vi "首页显示设置.vi"() -> ()   [LabVIEW 2016]
uses:
  <vilib>/Utility/miscctls.llb/LVPointTypeDef.ctl
  <vilib>/Utility/config.llb/NI_LVConfig.lvlib
panel:
  in  "CODCr":bool caption="氨氮禁用"
  in  "ORP":bool caption="氨氮禁用"
  in  "硫化物":bool caption="氨氮禁用"
  in  "亚硝氮":bool caption="氨氮禁用"
  in  "硝氮":bool caption="氨氮禁用"
  in  "确认":bool
  in  "藻密度":bool=TRUE caption="氨氮禁用"
  in  "叶绿素a":bool=TRUE caption="氨氮禁用"
  in  "湿度":bool=TRUE caption="氨氮禁用"
  in  "室温":bool=TRUE caption="氨氮禁用"
  in  "电压":bool=TRUE caption="氨氮禁用"
  in  "CODMn":bool=TRUE caption="氨氮禁用"
  in  "总氮":bool=TRUE caption="氨氮禁用"
  in  "总磷":bool=TRUE caption="氨氮禁用"
  in  "氨氮":bool=TRUE caption="氨氮禁用"
  in  "Turb":bool=TRUE caption="氨氮禁用"
  in  "Cond":bool=TRUE caption="氨氮禁用"
  in  "DO":bool=TRUE caption="氨氮禁用"
  in  "pH":bool=TRUE caption="氨氮禁用"
  in  "水温":bool=TRUE caption="氨氮禁用"
  # "请选择首页要显示的参数"
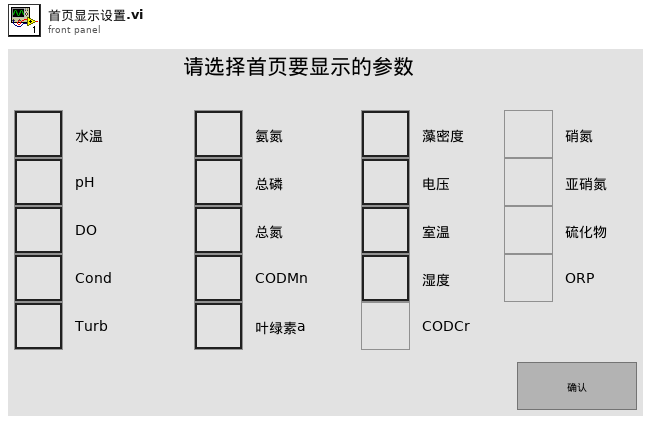
[diagram p1: front panel]
types:
  T1 = typedef "LVPointTypeDef.ctl" = cluster{"Horizontal":i16, "Vertical":i16}
  T2 = typedef "NI_LVConfig.lvlib/Config Data RefNum.ctl" = refnum<k1>
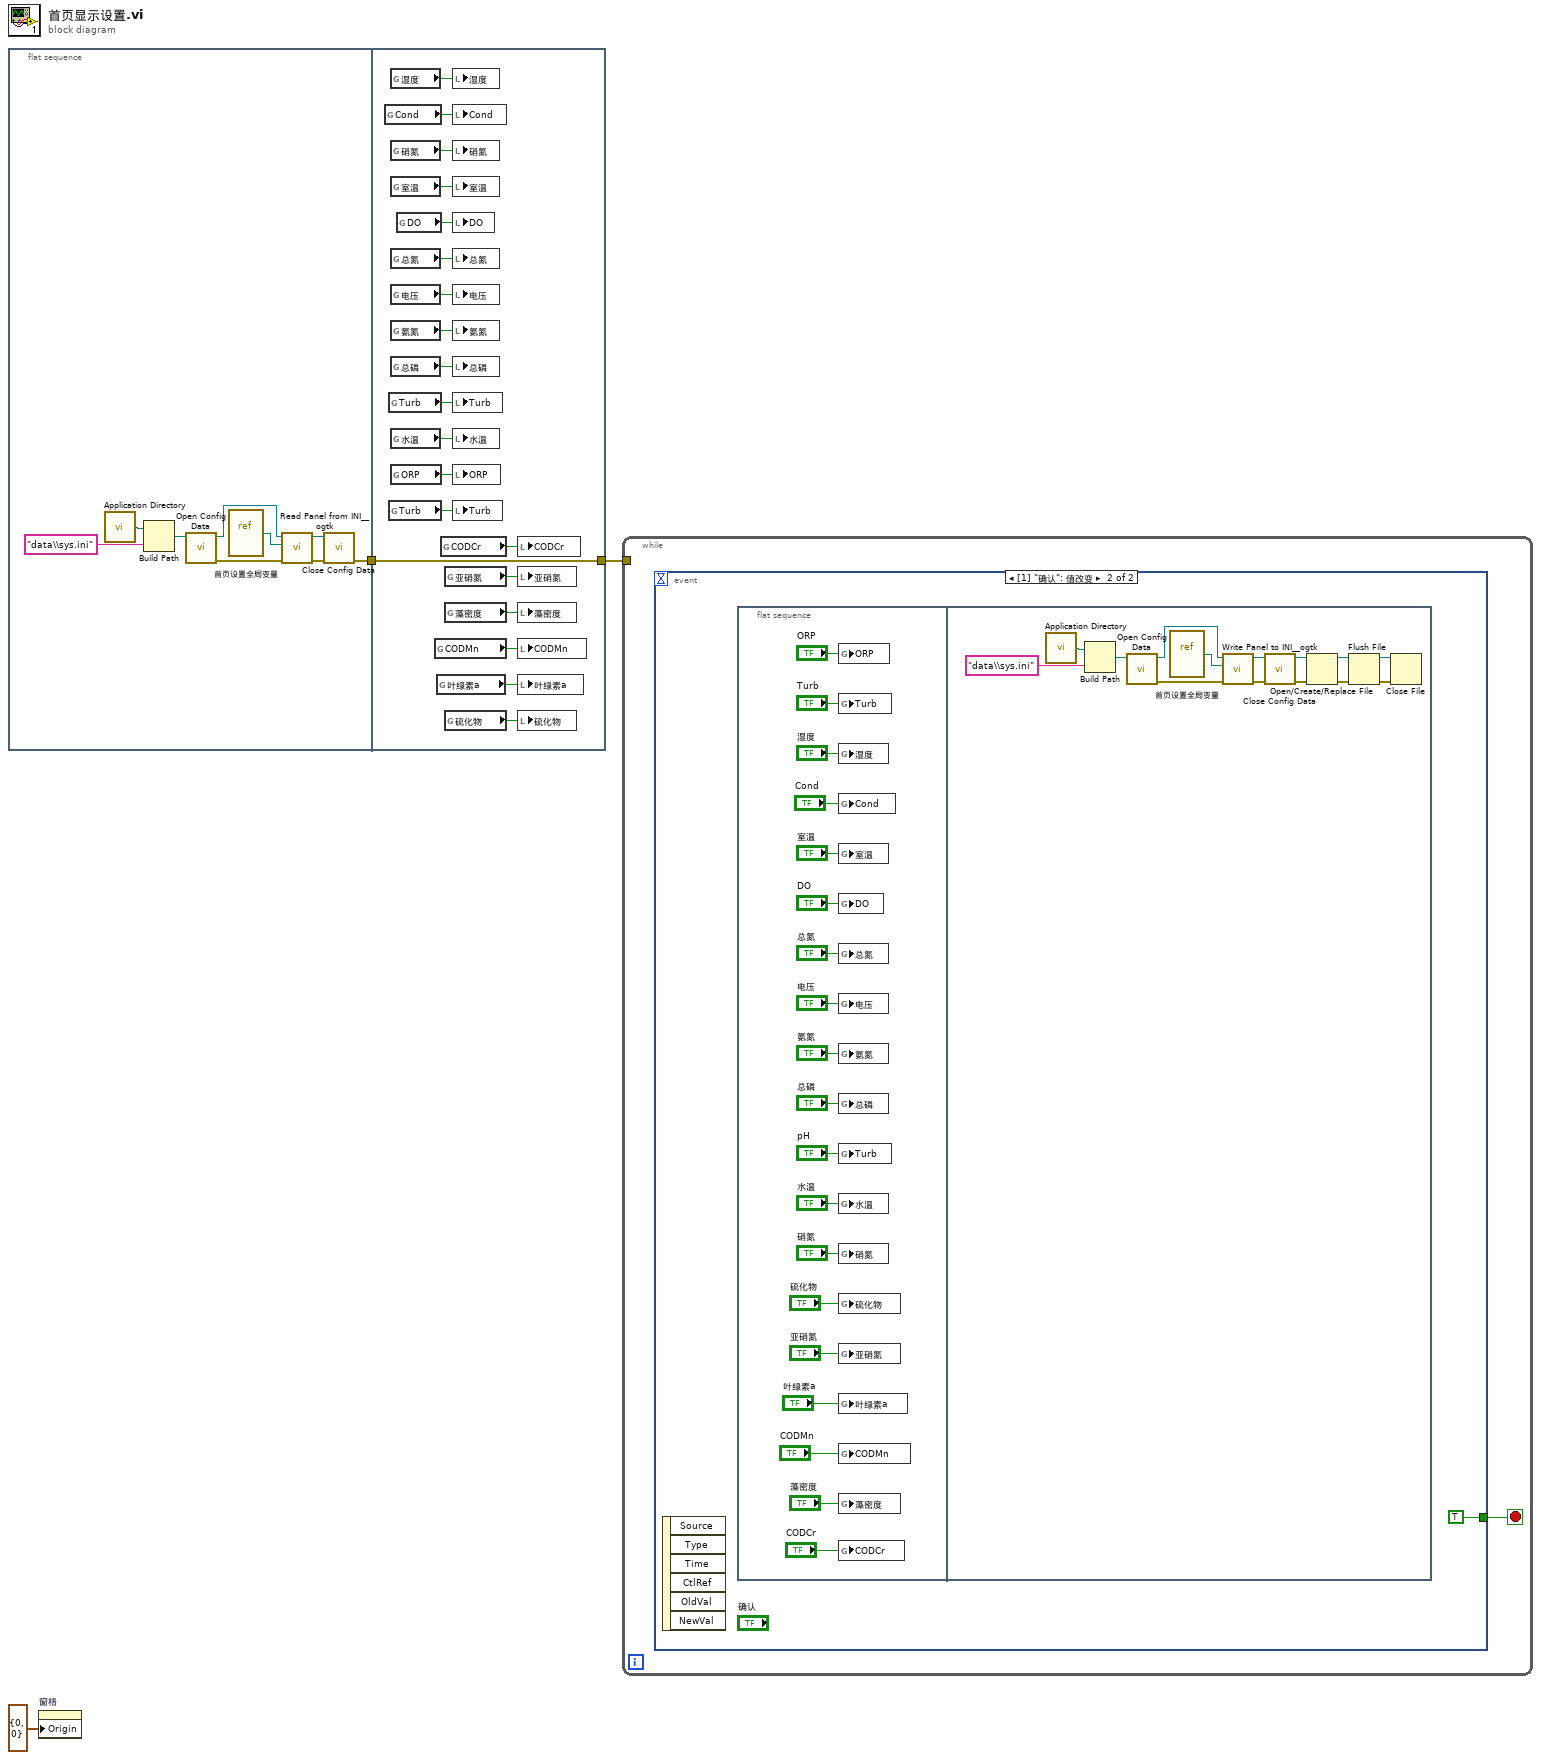
[diagram p0: block diagram]
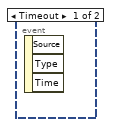
[diagram p2: hidden frame]
diagram:
  n1 = flat-sequence {
    tunnel: [w4] -> w2
    tunnel: w2 -> [w18]
    tunnel: [w18] -> w1
    frame #0 {
      n2 = call <vilib>:"Application Directory.vi"() -> ("Application Directory"=w12:path)
      n3 = Build Path(base path=w12, name or relative path="data\\sys.ini" ("名称或相对路径")) -> (appended path=w10:path)
      n4 = call <vilib>:"Open Config Data.vi"("configuration file path"=w10) -> ("error out"=w6:errorcluster, "refnum"=w9:T2)  [unwired: 8 in, 1 out]
      n5 = vi-ref "首页设置全局变量.vi"() -> (w8:refnum<vi>)
      n6 = call <userlib>:"Read Panel from INI__ogtk.vi"("error in (no error)"=w6, "VI ref"=w8, "refnum"=w9) -> ("error out"=w5:errorcluster, "refnum out"=w7:T2)  [unwired: 7 in]
      n7 = call <vilib>:"Close Config Data.vi"("error in (no error)"=w5, "refnum"=w7) -> ("error out"=w4:errorcluster)  [unwired: 8 in, 1 out]
    }
    frame #1 {
      n8 = global read "首页设置全局变量.vi" "Cond"() -> (w19:bool)
      n9 = global read "首页设置全局变量.vi" "Turb"() -> (w26:bool)
      n10 = global read "首页设置全局变量.vi" "Turb"() -> (w28:bool)
      n11 = global read "首页设置全局变量.vi" "湿度"() -> (w32:bool)
      n12 = global read "首页设置全局变量.vi" "硝氮"() -> (w17:bool)
      n13 = global read "首页设置全局变量.vi" "室温"() -> (w20:bool)
      n14 = global read "首页设置全局变量.vi" "总氮"() -> (w22:bool)
      n15 = global read "首页设置全局变量.vi" "电压"() -> (w23:bool)
      n16 = global read "首页设置全局变量.vi" "氨氮"() -> (w24:bool)
      n17 = global read "首页设置全局变量.vi" "总磷"() -> (w25:bool)
      n18 = global read "首页设置全局变量.vi" "水温"() -> (w27:bool)
      n19 = global read "首页设置全局变量.vi" "ORP"() -> (w14:bool)
      n20 = global read "首页设置全局变量.vi" "DO"() -> (w21:bool)
      n21 = global read "首页设置全局变量.vi" "CODMn"() -> (w30:bool)
      n22 = global read "首页设置全局变量.vi" "叶绿素a"() -> (w29:bool)
      n23 = global read "首页设置全局变量.vi" "CODCr"() -> (w13:bool)
      n24 = global read "首页设置全局变量.vi" "亚硝氮"() -> (w16:bool)
      n25 = global read "首页设置全局变量.vi" "藻密度"() -> (w31:bool)
      n26 = global read "首页设置全局变量.vi" "硫化物"() -> (w15:bool)
      n27 = local write "湿度"(w32) -> ()
      n28 = local write "Cond"(w19) -> ()
      n29 = local write "硝氮"(w17) -> ()
      n30 = local write "室温"(w20) -> ()
      n31 = local write "DO"(w21) -> ()
      n32 = local write "总氮"(w22) -> ()
      n33 = local write "电压"(w23) -> ()
      n34 = local write "氨氮"(w24) -> ()
      n35 = local write "总磷"(w25) -> ()
      n36 = local write "Turb"(w26) -> ()
      n37 = local write "水温"(w27) -> ()
      n38 = local write "ORP"(w14) -> ()
      n39 = local write "Turb"(w28) -> ()
      n40 = local write "CODCr"(w13) -> ()
      n41 = local write "亚硝氮"(w16) -> ()
      n42 = local write "藻密度"(w31) -> ()
      n43 = local write "CODMn"(w30) -> ()
      n44 = local write "叶绿素a"(w29) -> ()
      n45 = local write "硫化物"(w15) -> ()
    }
  }
  n46 = property on="窗格" class="Pane"("Origin"=T1 {"Horizontal"=0, "Vertical"=0} ("原点")) -> ()  [unwired: 2 in, 2 out]
  n47 = while {
    tunnel: w1 -> [_]
    stop <- w33 stop-if-true
    n48 = event shown="[1] \"确认\": 值改变" {
      selector: _ -> [_ _]
      dyn-events: _ -> [_ _]
      timeout: _ -> [_ _]
      tunnel: [_ TRUE] -> w33
      event Timeout {
        n49 = event-data() -> ()  [unwired: 1 in, 3 out]
      }
      event "确认": Value Change {
        n50 = event-data() -> ()  [unwired: 1 in, 6 out]
        n51 = flat-sequence {
          frame #0 {
            n52 = global write "首页设置全局变量.vi" "ORP"("ORP") -> ()
            n53 = global write "首页设置全局变量.vi" "Turb"("Turb") -> ()
            n54 = global write "首页设置全局变量.vi" "湿度"("湿度") -> ()
            n55 = global write "首页设置全局变量.vi" "Cond"("Cond") -> ()
            n56 = global write "首页设置全局变量.vi" "室温"("室温") -> ()
            n57 = global write "首页设置全局变量.vi" "DO"("DO") -> ()
            n58 = global write "首页设置全局变量.vi" "总氮"("总氮") -> ()
            n59 = global write "首页设置全局变量.vi" "电压"("电压") -> ()
            n60 = global write "首页设置全局变量.vi" "氨氮"("氨氮") -> ()
            n61 = global write "首页设置全局变量.vi" "总磷"("总磷") -> ()
            n62 = global write "首页设置全局变量.vi" "Turb"("pH") -> ()
            n63 = global write "首页设置全局变量.vi" "水温"("水温") -> ()
            n64 = global write "首页设置全局变量.vi" "硝氮"("硝氮") -> ()
            n65 = global write "首页设置全局变量.vi" "硫化物"("硫化物") -> ()
            n66 = global write "首页设置全局变量.vi" "亚硝氮"("亚硝氮") -> ()
            n67 = global write "首页设置全局变量.vi" "叶绿素a"("叶绿素a") -> ()
            n68 = global write "首页设置全局变量.vi" "CODMn"("CODMn") -> ()
            n69 = global write "首页设置全局变量.vi" "藻密度"("藻密度") -> ()
            n70 = global write "首页设置全局变量.vi" "CODCr"("CODCr") -> ()
          }
          frame #1 {
            n71 = call <vilib>:"Application Directory.vi"() -> ("Application Directory"=w54:path)
            n72 = Build Path(base path=w54, name or relative path="data\\sys.ini" ("名称或相对路径")) -> (appended path=w56:path)
            n73 = call <vilib>:"Open Config Data.vi"("configuration file path"=w56) -> ("error out"=w60:errorcluster, "refnum"=w57:T2)  [unwired: 8 in, 1 out]
            n74 = vi-ref "首页设置全局变量.vi"() -> (w58:refnum<vi>)
            n75 = call <userlib>:"Write Panel to INI__ogtk.vi"("error in (no error)"=w60, "VI ref"=w58, "refnum"=w57) -> ("error out"=w61:errorcluster, "refnum out"=w59:T2)  [unwired: 7 in]
            n76 = call <vilib>:"Close Config Data.vi"("error in (no error)"=w61, "refnum"=w59) -> ("error out"=w66:errorcluster, "file path"=w67:path)  [unwired: 8 in]
            n77 = Open/Create/Replace File(file path (use dialog)=w67, error in=w66) -> (refnum out=w63:refnum<file>, error out=w62:errorcluster)  [unwired: 4 in, 1 out]
            n78 = Flush File(refnum=w63, error in=w62) -> (refnum out=w64:refnum<file>, error out=w65:errorcluster)
            n79 = Close File(refnum=w64, error in=w65) -> ()  [unwired: 2 out]
          }
        }
      }
    }
  }
